vi "simple test.vi"() -> ()   [LabVIEW 2023]
uses:
  Measure and Stimulus Subsystems/Measure and Stimulus Subsystems.lvclass
panel:
  in  "Stop":bool
  out "Photosensor Waveform Chart":waveform(dbl)(graph)
  out "Error Out":errorcluster
  out "Powersensor Scalar":dbl
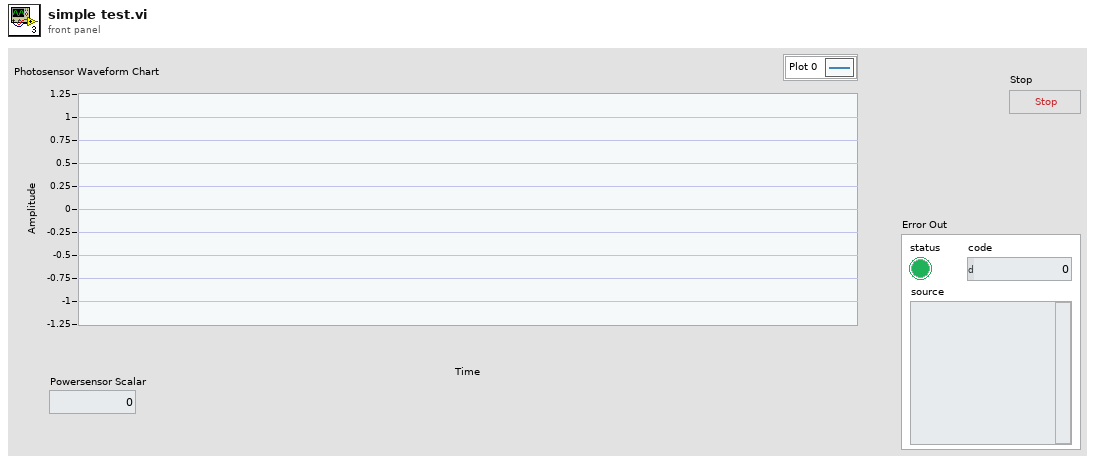
[diagram p1: front panel]
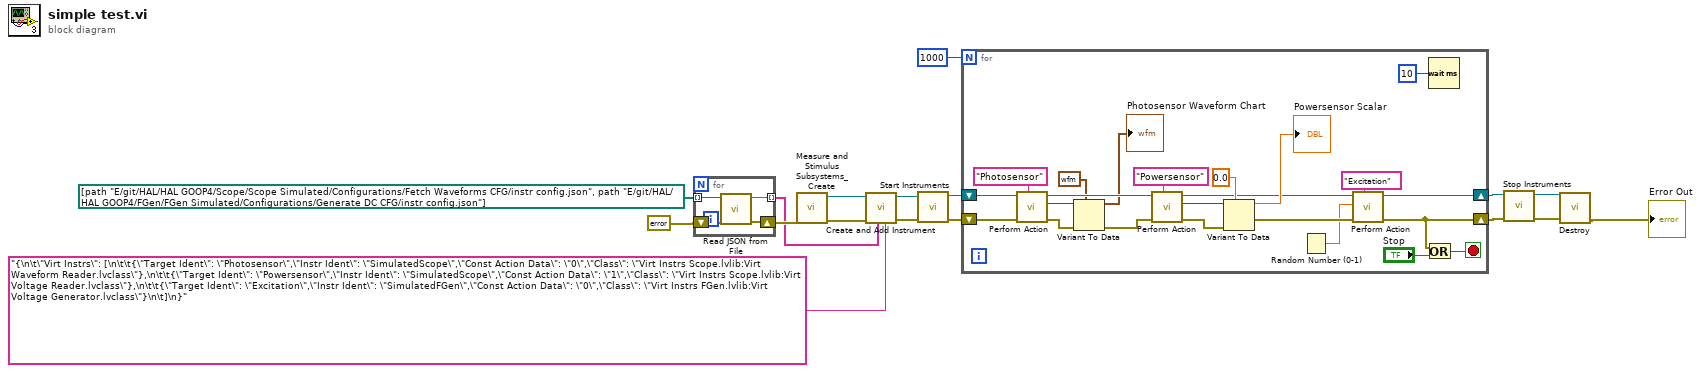
[diagram p0: block diagram]
diagram:
  n1 = for {
    tunnel: path[] [path "E:/git/HAL/HAL GOOP4/Scope/Scope Simulated/Configurations/Fetch Waveforms CFG/instr config.json", path "E:/git/HAL/HAL GOOP4/FGen/FGen Simulated/Configurations/Generate DC CFG/instr config.json"] -> [w21] mode=indexing
    shift-right: [w19] -> w4
    shift-left: errorcluster {"status"=FALSE, "code"=0, "source"=""} ("error out") -> [w20]
    tunnel: [w18] -> w3 mode=indexing
    n2 = call "Read JSON from File.vi"("error in (no error)"=w20, "File Path"=w21) -> ("error out"=w19:errorcluster, "<JSON>Config"=w18:string)  [unwired: 8 in]
  }
  n3 = call "Measure and Stimulus Subsystems_Create.vi"("Error In"=w4) -> ("Error Out"=w16:errorcluster, "reference out"=w17:refnum<class "Measure and Stimulus Subsystems.lvclass">)  [unwired: 9 in]
  n4 = call-dynamic "Create and Add Instrument.vi"("Virt Instr JSON Config"="{\n\t\"Virt Instrs\": [\n\t\t{\"Target Ident\": \"Photosensor\",\"Instr Ident\": \"SimulatedScope\",\"Const Action Data\": \"0\",\"Class\": \"Virt Instrs Scope.lvlib:Virt Waveform Reader.lvclass\"},\n\t\t{\"Target Ident\": \"Powersensor\",\"Instr Ident\": \"SimulatedScope\",\"Const Action Data\": \"1\",\"Class\": \"Virt Instrs Scope.lvlib:Virt Voltage Reader.lvclass\"},\n\t\t{\"Target Ident\": \"Excitation\",\"Instr Ident\": \"SimulatedFGen\",\"Const Action Data\": \"0\",\"Class\": \"Virt Instrs FGen.lvlib:Virt Voltage Generator.lvclass\"}\n\t]\n}", "Physical Intr Configs"=w3, "Error In"=w16, "reference in"=w17) -> ("Error Out"=w15:errorcluster, "reference out"=w13:refnum<class "Measure and Stimulus Subsystems.lvclass">)  [unwired: 6 in]
  n5 = call "Start Instruments.vi"("Error In"=w15, "reference in"=w13) -> ("Error Out"=w14:errorcluster, "reference out"=w12:refnum<class "Measure and Stimulus Subsystems.lvclass">)  [unwired: 8 in]
  n6 = for {
    N: 1000 -> [_]
    shift-right: [w26] -> w7
    shift-left: w14 -> [w39]
    shift-right: [w24] -> w10
    shift-left: w12 -> [w38]
    stop <- w27 stop-if-true
    n7 = call "Perform Action.vi"("Target Ident"="Photosensor" ("Target Identifier"), "Error In"=w39, "reference in"=w38) -> ("Error Out"=w42:errorcluster, "Output"=w36:variant, "reference out"=w43:refnum<class "Measure and Stimulus Subsystems.lvclass">)  [unwired: 6 in]
    n8 = Variant To Data(error in=w42, type=waveform(dbl) {"t0"=timestamp(0 s since 1904-01-01), "dt"=1.0, "Y"=[]} ("Waveform"), Variant=w36) -> (data=→"Photosensor Waveform Chart":waveform(dbl), error out=w37:errorcluster)
    n9 = call "Perform Action.vi"("Target Ident"="Powersensor" ("Target Identifier"), "Error In"=w37, "reference in"=w43) -> ("Error Out"=w40:errorcluster, "Output"=w34:variant, "reference out"=w25:refnum<class "Measure and Stimulus Subsystems.lvclass">)  [unwired: 6 in]
    n10 = Variant To Data(error in=w40, type=0.0, Variant=w34) -> (data=→"Powersensor Scalar":dbl, error out=w28:errorcluster)
    n11 = Random Number (0-1)() -> (number: 0 to 1=w22:dbl)
    n12 = call "Perform Action.vi"("Target Ident"="Excitation", "Error In"=w28, "Input"=w22, "reference in"=w25) -> ("Error Out"=w26:errorcluster, "reference out"=w24:refnum<class "Measure and Stimulus Subsystems.lvclass">)  [unwired: 5 in, 1 out]
    n13 = Or(x=w26, y="Stop") -> (x .or. y?=w27:bool)
    n14 = Wait (ms)(milliseconds to wait=u32 10) -> ()  [unwired: 1 out]
  }
  n15 = call "Stop Instruments.vi"("Error In"=w7, "reference in"=w10) -> ("Error Out"=w11:errorcluster, "reference out"=w9:refnum<class "Measure and Stimulus Subsystems.lvclass">)  [unwired: 8 in]
  n16 = call-dynamic "Destroy.vi"("Error In"=w11, "reference in"=w9) -> ("Error Out"=→"Error Out":errorcluster)  [unwired: 8 in, 1 out]
